vi "SUB_Write Characters To File.vi"(0 "convert eol? (no:F)":bool caption="eol 변환? (아니오:거짓)", 3 "append to file? (new file:F)":bool caption="파일에 추가? (새 파일:거짓)", 4 "character string":string caption="문자 문자열", 5 "file path (dialog if empty)":path caption="파일 경로(비었을 경우 대화 상자)") -> (2 "new file path (Not A Path if cancelled)":path caption="새 파일 경로(취소될 경우 경로 없음)")   [LabVIEW 2015]
doc: "LabVIEW는 더 이상 이 VI를 지원하지 않습니다. 대신에 [텍스트 파일에 쓰기] 함수를 사용하십시오. <B>문자 문자열</B>을 새 바이트 스트림 파일에 쓰거나 문자열을 기존의 파일에 추가합니다. VI는 쓰기 전에 파일을 열거나 생성하고 쓴 후에 파일을 닫습니다."
panel:
  in  "prompt":string="쓸 파일을 선택하십시오." caption="입력요청"
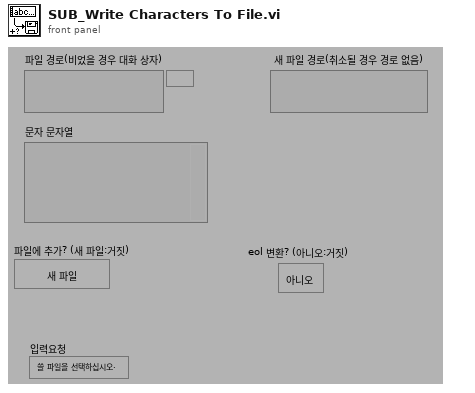
[diagram p1: front panel]
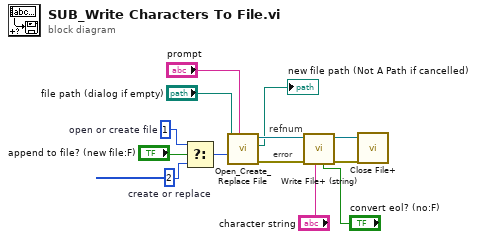
[diagram p0: block diagram]
diagram:
  w5 = i16 2  # create or replace
  w8 = i16 1  # open or create file
  # "error"
  # "refnum"
  n1 = Select(t=w8, s="append to file? (new file:F)", f=w5) -> (s? t:f=w9:i16)
  n2 = call <vilib>:"Open_Create_Replace File.vi"("prompt"="prompt", "function (open:0)"=w9, "file path"="file path (dialog if empty)") -> ("error out"=w12:errorcluster, "new file path"=→"new file path (Not A Path if cancelled)":path, "refnum"=w4:refnum<file>)  [unwired: 5 in, 1 out]
  n3 = call <vilib>:"Write File+ (string).vi"("convert eol? (no:F)"="convert eol? (no:F)", "string"="character string", "error in (no error)"=w12, "refnum"=w4) -> ("error out"=w11:errorcluster, "dup refnum"=w10:refnum<file>)  [unwired: 3 in, 1 out]
  n4 = call <vilib>:"Close File+.vi"("error in (no error)"=w11, "refnum"=w10) -> ()  [unwired: 3 in, 3 out]
